vi "UI_updateUI.vi"(6 "UI_controlRefs":T3, 8 "error in (no error)":errorcluster, 9 "Player Winnings":refnum<vi>[](array[refnum]), 10 "Player LEDs":refnum<vi>[](array[refnum]), 11 "Game State":T1) -> (0 "error out":errorcluster, 3 "Game State OUT":T1)   [LabVIEW 2020]
uses:
  Typedefs/gameState.ctl
  Typedefs/enumeratedPlayers.ctl
  Typedefs/UI_controlRefs.ctl
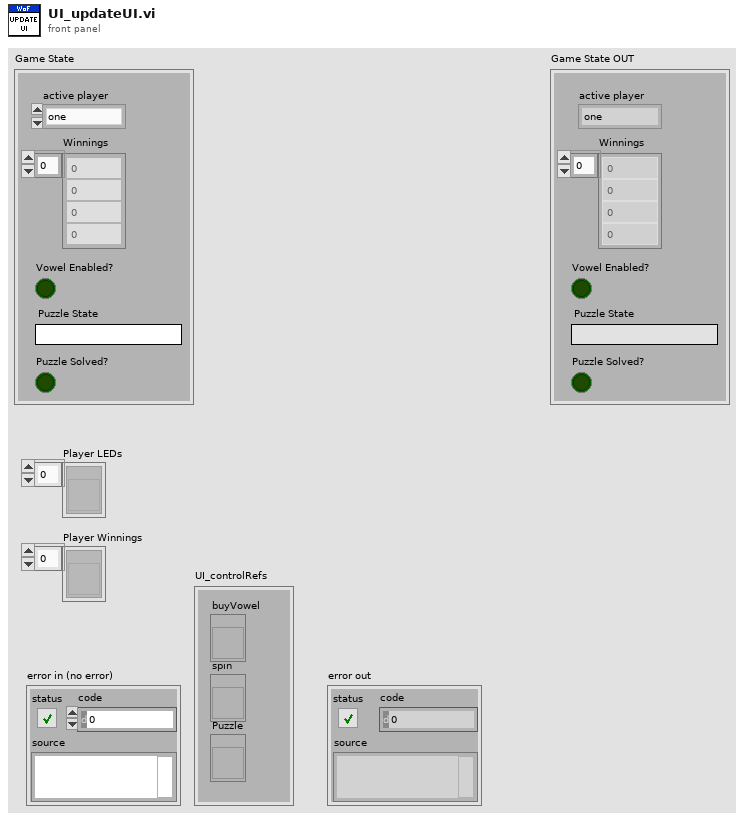
[diagram p1: front panel]
types:
  T1 = typedef "gameState.ctl" = cluster{"active player":T2, "Winnings":dbl[], "Vowel Enabled?":bool, "Puzzle State":string, "Puzzle Solved?":bool}
  T2 = typedef "enumeratedPlayers.ctl" = enum16{"one", "two", "three"}
  T3 = typedef "UI_controlRefs.ctl" = cluster{"spin":refnum<vi>, "buyVowel":refnum<vi>, "Puzzle":refnum<vi>}
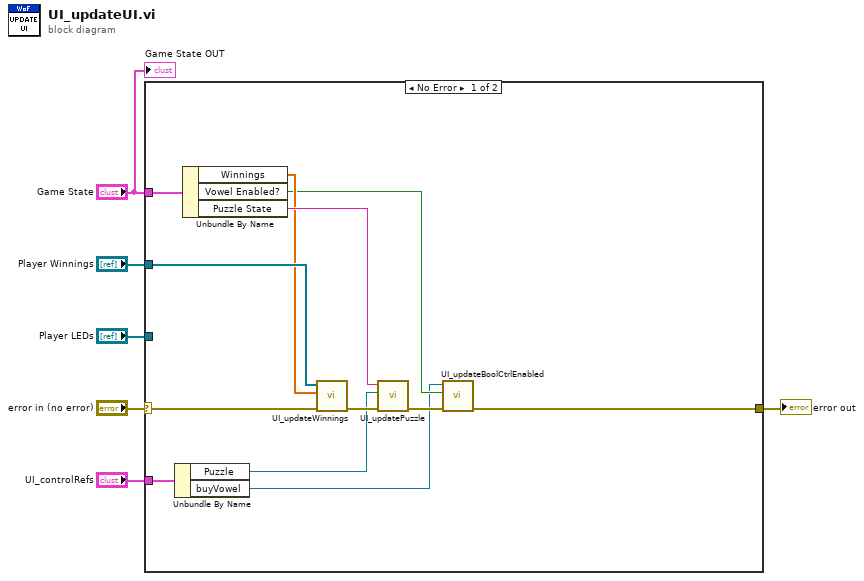
[diagram p0: block diagram]
diagram:
  n1 = case shown="No Error" "error in (no error)" {
    selector: "error in (no error)" -> [w16 w19]
    tunnel: "Game State" -> [w17 _]
    tunnel: "Player Winnings" -> [w15 _]
    tunnel: "Player LEDs" -> [_ _]
    tunnel: "UI_controlRefs" -> [w18 _]
    tunnel: [w7 w19] -> w1
    frame No Error {
      n2 = Unbundle By Name(w18) -> ("Puzzle"=w13:refnum<vi>, "buyVowel"=w8:refnum<vi>)
      n3 = Unbundle By Name(w17) -> ("Winnings"=w10:dbl[], "Vowel Enabled?"=w9:bool, "Puzzle State"=w12:string)
      n4 = call "UI_updateWinnings.vi"("error in (no error)"=w16, "Winnings"=w10, "Numeric Controls"=w15) -> ("error out"=w14:errorcluster)  [unwired: 8 in]
      n5 = call "UI_updatePuzzle.vi"("error in (no error)"=w14, "Puzzle"=w13, "Puzzle state"=w12) -> ("error out"=w11:errorcluster)  [unwired: 8 in]
      n6 = call "UI_updateBoolCtrlEnabled.vi"("error in (no error)"=w11, "Enabled?"=w9, "boolRef"=w8) -> ("error out"=w7:errorcluster)  [unwired: 8 in]
    }
    frame Error {
    }
  }
  "error out" <- w1
  "Game State OUT" <- "Game State"
